vi "Exp_ICCD_SetGateMode.vi"(8 "error in (no error)":errorcluster, 10 "Gate Mode":string(combo)="Repetitive", 11 "LightField Automation in":refnum<class "LightField Automation.lvclass">) -> (0 "error out":errorcluster, 3 "LightField Automation out":refnum<class "LightField Automation.lvclass">)   [LabVIEW 2019, in "LightField Automation.lvclass"]
uses:
  LightField Automation.lvclass
  C:/Program Files/Princeton Instruments/LightField/PrincetonInstruments.LightFieldAddInSupportServices.dll
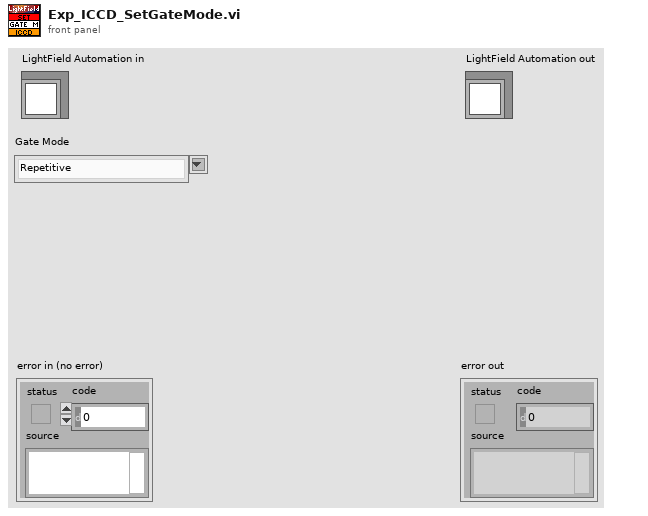
[diagram p1: front panel]
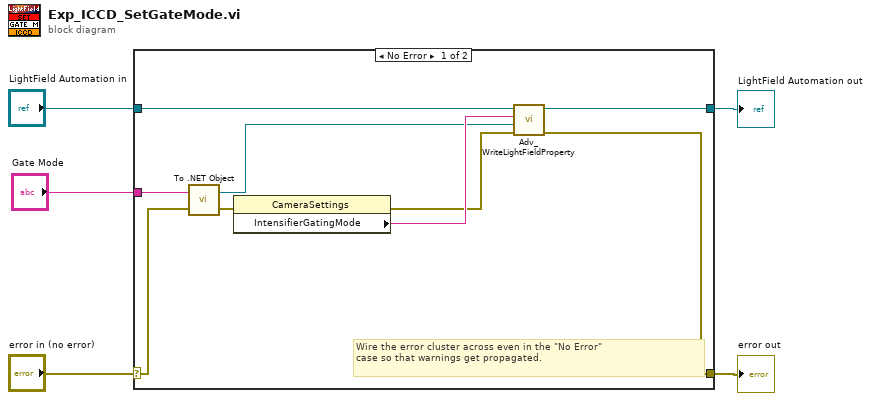
[diagram p0: block diagram]
diagram:
  n1 = case shown="No Error" "error in (no error)" {
    selector: "error in (no error)" -> [w13 w16]
    tunnel: [w6 w16] -> w4
    tunnel: [w11 w15] -> w2
    tunnel: "LightField Automation in" -> [w10 w15]
    tunnel: "Gate Mode" -> [w14 _]
    frame No Error {
      # "Wire the error cluster across even in the \"No Error\"\ncase so that warnings get propagated."
      n2 = call <vilib>:"To .NET Object.vi"("error in (no error)"=w13, "anything"=w14) -> ("error out"=w12:errorcluster, ".NET object"=w7:refnum<k24>)
      n3 = property class="CameraSettings"(error in=w12) -> (error out=w8:errorcluster, "IntensifierGatingMode"=w9:string)  [unwired: 1 in, 1 out]
      n4 = call "Adv_WriteLightFieldProperty.vi"("error in (no error)"=w8, "value"=w7, "setting"=w9, "LightField Automation in"=w10) -> ("error out"=w6:errorcluster, "LightField Automation out"=w11:refnum<class "LightField Automation.lvclass">)  [unwired: 6 in]
    }
    frame Error {
    }
  }
  "error out" <- w4
  "LightField Automation out" <- w2
